vi "Read analog voltage on slow analog input.vi"() -> ()   [LabVIEW 2017]
doc: "This example shows how to measure analog voltage of slow analog inputs on Red Pitaya extension connector. Analog inputs on Red Pitaya are rated from 0-3.3 Volts."
uses:
  RedPitaya.lvlib
panel:
  out "Voltage":dbl
  in  "Pin Name":string="AIN3"
  out "LEDs":bool[](array[boolean])
  in  "IP address":string="192.168.4.129"
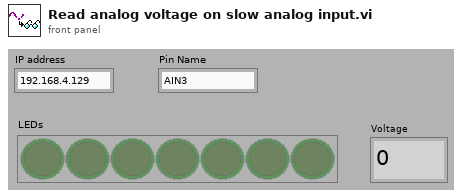
[diagram p1: front panel]
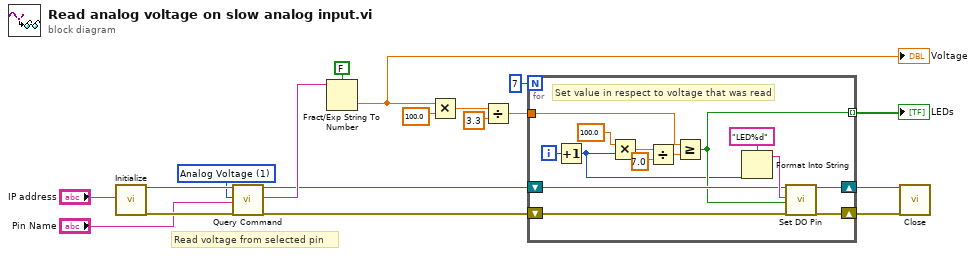
[diagram p0: block diagram]
diagram:
  w15 = u16 1 items=["State of Digital IOs", "Analog Voltage", "Decimation", "Sampling Rate", "Sampling Rate (Hz)", "Averaging Status", "Trigger Status", "Trigger Delay in Samples", "Trigger Delay in Nanoseconds", "Trigger Level in mV", "Current Position of Write Pointer", "Position of Trigger Event", "Buffer Size"] ("Query setting")
  # "Read voltage from selected pin"
  n1 = call "Initialize.vi"("IP address"="IP address") -> ("RedPitaya connection out"=w17:refnum<k5>, "error out"=w16:errorcluster)  [unwired: 17 in]
  n2 = call "Query Command.vi"("RedPitaya connection in"=w17, "Query setting"=w15, "Pin Name"="Pin Name", "error in"=w16) -> ("RedPitaya connection out"=w11:refnum<k5>, "Output string"=w14:string, "error out"=w12:errorcluster)  [unwired: 13 in]
  n3 = Fract/Exp String To Number(use system decimal point (T)=FALSE, string=w14) -> (number=w2:dbl)  [unwired: 2 in, 1 out]
  "Voltage" <- w2
  n4 = Multiply(x=w2, y=100.0) -> (x*y=w9:dbl)
  n5 = Divide(x=w9, y=3.3) -> (x/y=w7:dbl)
  n6 = for {
    N: 7 -> [_]
    tunnel: w7 -> [w28]
    shift-right: [w22] -> w6
    shift-left: w11 -> [w23]
    shift-right: [w21] -> w5
    shift-left: w12 -> [w24]
    tunnel: [w20] -> w4 mode=indexing
    i -> [w26]
    # "Set value in respect to voltage that was read"
    n7 = Increment(x=w26) -> (x+1=w19:i32)
    n8 = Multiply(x=100.0, y=w19) -> (x*y=w30:dbl)
    n9 = Divide(x=w30, y=7.0) -> (x/y=w32:dbl)
    n10 = Greater Or Equal?(x=w28, y=w32) -> (x >= y?=w20:bool)
    n11 = Format Into String(format string="LED%d", w19) -> (resulting string=w25:string)  [unwired: 2 in, 1 out]
    n12 = call "Set DO Pin.vi"("RedPitaya connection in"=w23, "Pin name"=w25, "State"=w20, "error in"=w24) -> ("RedPitaya connection out"=w22:refnum<k5>, "error out"=w21:errorcluster)  [unwired: 14 in]
  }
  "LEDs" <- w4
  n13 = call "Close.vi"("RedPitaya connection in"=w6, "error in"=w5) -> ()  [unwired: 17 in, 1 out]
